vi "modify_build_number.vi"(11 "args":string[](array[string])) -> (2 "error":string, 3 "code":i32)   [LabVIEW 2017]
uses:
  <vilib>/AppBuilder/AB_API_Simple/Build Specification Version.ctl
  <vilib>/AppBuilder/AB_API_Simple/Set Build Specification Version (path).vi
  <vilib>/AppBuilder/AB_API_Simple/NI_App_Builder_API.lvlib
panel:
  in  "error in (no error)":errorcluster
  out "error out":errorcluster
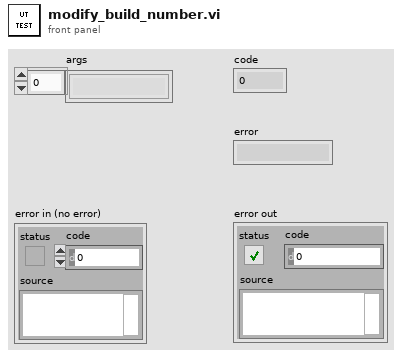
[diagram p1: front panel]
types:
  T1 = typedef "NI_App_Builder_API.lvlib/Build Specification Version.ctl" = cluster{"Major":u16, "Minor":u16, "Fix":u16, "Build":u16}
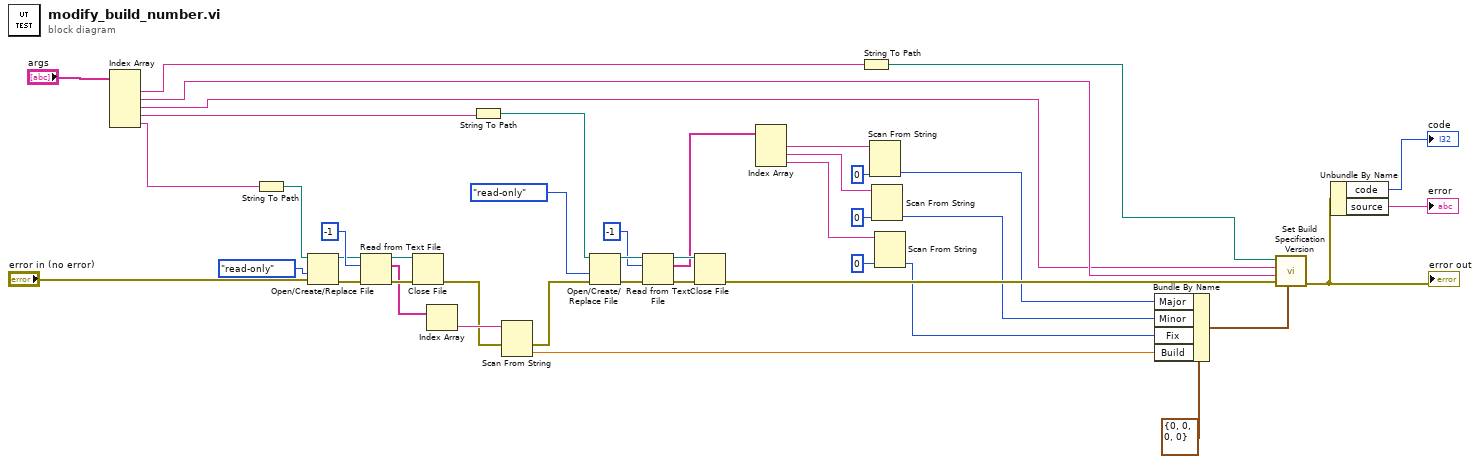
[diagram p0: block diagram]
diagram:
  n1 = Index Array(array="args") -> (element #1=w7:string, element #2=w6:string, element #3=w5:string, element #4=w33:string, element #5=w19:string)  [unwired: 5 in]
  n2 = String To Path(string=w19) -> (path=w18:path)
  n3 = Open/Create/Replace File(file path (use dialog)=w18, error in="error in (no error)", access (0:read/write)=enum16{"read/write", "read-only", "write-only"}."read-only") -> (refnum out=w26:refnum<file>, error out=w27:errorcluster)  [unwired: 3 in, 1 out]
  n4 = Read from Text File(file (use dialog)=w26, count=-1, error in=w27) -> (refnum out=w29:refnum<file>, text=w23:string[], error out=w30:errorcluster)  [unwired: 1 in, 1 out]
  n5 = Close File(refnum=w29, error in=w30) -> (error out=w22:errorcluster)  [unwired: 1 out]
  n6 = Index Array(array=w23) -> (element=w31:string)  [unwired: 1 in]
  n7 = String To Path(string=w33) -> (path=w32:path)
  n8 = Scan From String(input string=w31, error in=w22) -> (error out=w21:errorcluster, output 1=w20:dbl)  [unwired: 3 in, 2 out]
  n9 = Open/Create/Replace File(file path (use dialog)=w32, error in=w21, access (0:read/write)=enum16{"read/write", "read-only", "write-only"}."read-only") -> (refnum out=w39:refnum<file>, error out=w38:errorcluster)  [unwired: 3 in, 1 out]
  n10 = Read from Text File(file (use dialog)=w39, count=-1, error in=w38) -> (refnum out=w36:refnum<file>, text=w11:string[], error out=w35:errorcluster)  [unwired: 1 in, 1 out]
  n11 = Close File(refnum=w36, error in=w35) -> (error out=w10:errorcluster)  [unwired: 1 out]
  n12 = Index Array(array=w11) -> (element #1=w17:string, element #2=w14:string, element #3=w12:string)  [unwired: 3 in]
  n13 = String To Path(string=w7) -> (path=w4:path)
  n14 = Scan From String(input string=w17, default 1=u16 0 ("Major")) -> (output 1=w3:u16)  [unwired: 3 in, 3 out]
  n15 = Scan From String(input string=w14, default 1=u16 0 ("Major")) -> (output 1=w2:u16)  [unwired: 3 in, 3 out]
  n16 = Scan From String(input string=w12, default 1=u16 0 ("Major")) -> (output 1=w1:u16)  [unwired: 3 in, 3 out]
  n17 = Bundle By Name(cluster=T1 {"Major"=0, "Minor"=0, "Fix"=0, "Build"=0} ("Build Specification Version"), "Major"=w3, "Minor"=w2, "Fix"=w1, "Build"=w20) -> (w9:T1)
  n18 = call-poly <vilib>:"Set Build Specification Version.vi"("Build Specification Version"=w9, "error in (no error)"=w10, "Name of target (My Computer)"=w6, "Name of build specification"=w5, "Path to project"=w4) -> ("error out"=w41:errorcluster)  [unwired: 6 in]
  "error out" <- w41
  n19 = Unbundle By Name(w41) -> ("code"=→"code":i32, "source"=→"error":string)
